vi "ImClass_Dataset_Reader.vi"(5 "Unique labels":string[](array[string]), 7 "Dims(C,H,W)":T1, 8 "error in (no error)":errorcluster, 11 "Image Foldr Path":path) -> (0 "error out":errorcluster, 3 "NN_DataSet(In3D_OutBBox)":T2)   [LabVIEW 2020]
uses:
  <vilib>/Ngene/Deep Learning Toolkit/Toolkit/NN_Data/API/DataSet/DataSet_Types/NN_DataSet(In3D_Out1D).ctl
  <vilib>/Ngene/Deep Learning Toolkit/Toolkit/NN_Data/Controls/DataRef_Types/2D/NN_Data_ref(2D_SGL).ctl
  <vilib>/Ngene/Deep Learning Toolkit/Toolkit/NN_Data/API/NN_Dims(C,H,W).ctl
  <vilib>/Ngene/Deep Learning Toolkit/Toolkit/Deep_Learning_Toolkit_by_Ngene.lvlib
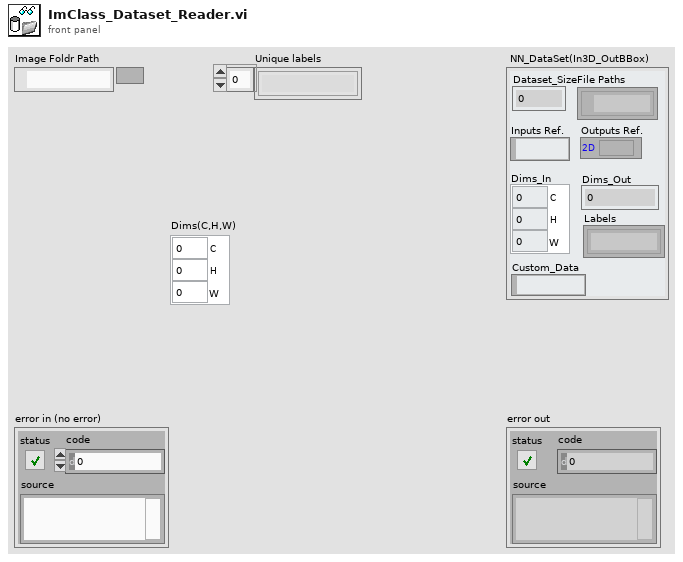
[diagram p1: front panel]
types:
  T1 = typedef "Deep_Learning_Toolkit_by_Ngene.lvlib/NN_Dims(C,H,W).ctl" = cluster{"C":i32, "H":i32, "W":i32}
  T2 = typedef "Deep_Learning_Toolkit_by_Ngene.lvlib/NN_DataSet(In3D_Out1D).ctl" = cluster{"Inputs Ref.":variant, "Outputs Ref.":T3, "Dataset_Size":i32, "Dims_In":T1, "Dims_Out":i32, "Labels":string[], "File Paths":path[], "Custom_Data":variant}
  T3 = typedef "Deep_Learning_Toolkit_by_Ngene.lvlib/NN_Data_ref(2D_SGL).ctl" = refnum<data-value>
  T4 = typedef "Image Type" = u32
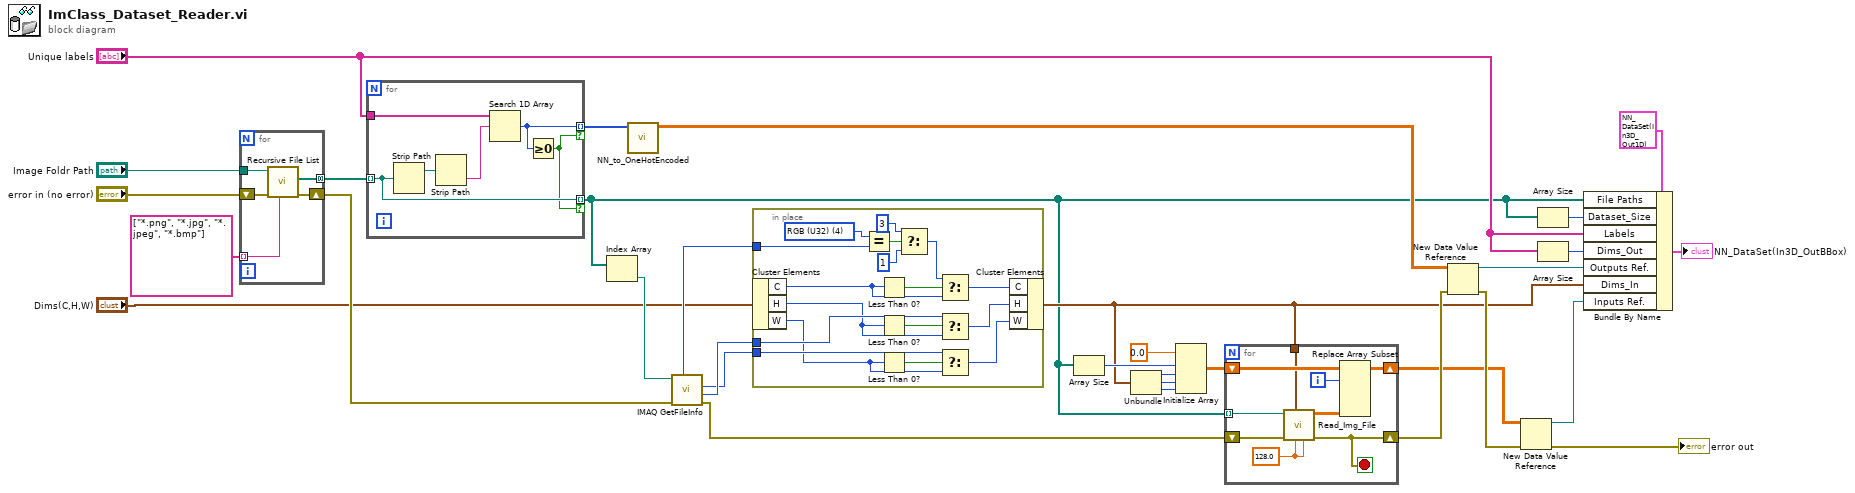
[diagram p0: block diagram]
diagram:
  n1 = for {
    tunnel: "Image Foldr Path" -> [w37]
    tunnel: string[] ["*.png", "*.jpg", "*.jpeg", "*.bmp"] ("pattern") -> [w36] mode=indexing
    tunnel: [w35] -> w30 mode=concatenating
    shift-right: [w33] -> w9
    shift-left: "error in (no error)" -> [w34]
    n2 = call <vilib>:"Recursive File List.vi"("pattern"=w36, "error in (no error)"=w34, "Folder Path"=w37) -> ("error out"=w33:errorcluster, "All Files in Dir"=w35:path[])  [unwired: 4 in, 3 out]
  }
  n3 = for {
    tunnel: w30 -> [w39] mode=indexing
    tunnel: "Unique labels" -> [w42]
    tunnel: [w40] -> w21 mode=indexing if=w38
    tunnel: [w39] -> w2 mode=indexing if=w38
    n4 = Strip Path(path=w39) -> (stripped path=w43:path)  [unwired: 1 out]
    n5 = Strip Path(path=w43) -> (name=w41:string)  [unwired: 1 out]
    n6 = Search 1D Array(1D array=w42, element=w41) -> (index of element=w40:i32)  [unwired: 1 in]
    n7 = Greater Or Equal To 0?(x=w40) -> (x >= 0?=w38:bool)
  }
  n8 = Index Array(array=w2) -> (element=w10:path)  [unwired: 1 in]
  n9 = call <vilib>:"NN_to_OneHotEncoded.vi"("Label_Idx"=w21) -> ("Prediction"=w22:sgl[][])  [unwired: 10 in]
  n10 = call "IMAQ GetFileInfo"("error in (no error)"=w9, "File Path"=w10) -> ("error out"=w8:errorcluster, "Y Resolution"=w7:i32, "X Resolution"=w6:i32, "Image Type"=w4:T4)  [unwired: 3 in, 3 out]
  n11 = in-place {
    in-place-border: w7 -> [w60]
    in-place-border: w6 -> [w59]
    in-place-border: w4 -> [w49]
    w48 = T4 4 items=["Grayscale (U8)", "Grayscale (I16)", "Grayscale (SGL)", "Complex (CSG)", "RGB (U32)", "HSL (U32)", "RGB (U64)", "Grayscale (U16)"] ("x")
    n12 = in-place-cluster #1("Dims(C,H,W)") -> ("C"=w55:i32, "H"=w54:i32, "W"=w44:i32)
    n13 = Equal?(x=w48, y=w49) -> (x = y?=w50:bool)
    n14 = Less Than 0?(x=w55) -> (x < 0?=w56:bool)
    n15 = Less Than 0?(x=w54) -> (x < 0?=w58:bool)
    n16 = Less Than 0?(x=w44) -> (x < 0?=w57:bool)
    n17 = Select(t=3 ("H"), s=w50, f=1 ("H")) -> (s? t:f=w45:i32)
    n18 = Select(t=w45, s=w56, f=w55) -> (s? t:f=w53:i32)
    n19 = Select(t=w60, s=w58, f=w54) -> (s? t:f=w52:i32)
    n20 = Select(t=w59, s=w57, f=w44) -> (s? t:f=w51:i32)
    n21 = in-place-cluster #1("C"=w53, "H"=w52, "W"=w51) -> (w5:T1)
  }
  n22 = Array Size(array=w2) -> (size(s)=w14:i32)
  n23 = Unbundle(w5) -> ("C"=w13:i32, "H"=w12:i32, "W"=w11:i32)
  n24 = Initialize Array(sgl 0.0 ("element"), w14, w13, w12, w11) -> (w18:sgl[][][][])
  n25 = for {
    tunnel: w2 -> [w62] mode=indexing
    shift-right: [w68] -> w16
    shift-left: w18 -> [w69]
    tunnel: w5 -> [w65]
    shift-right: [w64] -> w24
    shift-left: w8 -> [w66]
    i -> [w67]
    stop <- w64 stop-if-true
    w61 = sgl 128.0 ("Shift")
    n26 = call "Read_Img_File.vi"("Divider"=w61, "Shift"=w61, "Dims(C,H,W)"=w65, "error in (no error)"=w66, "Path"=w62) -> ("error out"=w64:errorcluster, "Data"=w63:sgl[][][])  [unwired: 3 in, 2 out]
    n27 = Replace Array Subset(array=w69, new element=w63, index (dim 0)=w67) -> (w68:sgl[][][][])  [unwired: 3 in]
  }
  n28 = New Data Value Reference(data value=w22, error in=w24) -> (data value reference=w23:refnum<data-value>, error out=w25:errorcluster)
  n29 = New Data Value Reference(data value=w16, error in=w25) -> (data value reference=w17:refnum<data-value>, error out=→"error out":errorcluster)
  n30 = Array Size(array=w2) -> (size(s)=w1:i32)
  n31 = Array Size(array="Unique labels") -> (size(s)=w15:i32)
  n32 = Bundle By Name(cluster=T2 {"Inputs Ref."=variant, "Outputs Ref."=refnum, "Dataset_Size"=0, "Dims_In"={"C"=0, "H"=0, "W"=0}, "Dims_Out"=0, "Labels"=[], "File Paths"=[], "Custom_Data"=variant} ("Dataset(In3D_Out1D)"), "File Paths"=w2, "Dataset_Size"=w1, "Labels"="Unique labels", "Dims_Out"=w15, "Outputs Ref."=w23, "Dims_In"=w5, "Inputs Ref."=w17) -> (→"NN_DataSet(In3D_OutBBox)":T2)
